vi "Day08-1.vi"() -> ()   [LabVIEW 2021]
panel:
  out "Numeric":i32
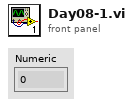
[diagram p1: front panel]
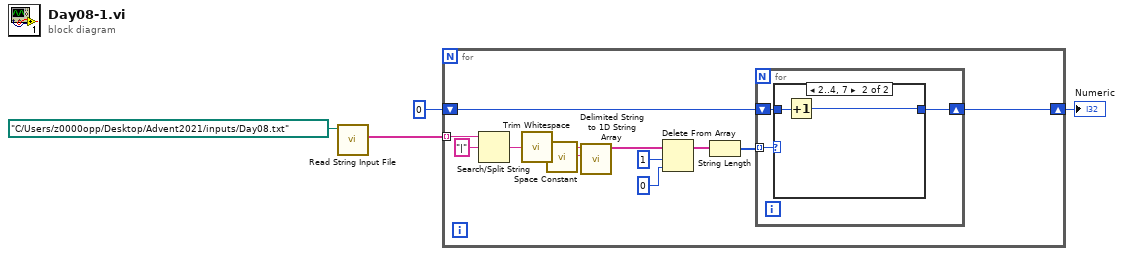
[diagram p0: block diagram]
diagram:
  n1 = call "Read String Input File.vi"("file path (dialog if empty)"=path "C:/Users/z0000opp/Desktop/Advent2021/inputs/Day08.txt") -> ("input values"=w3:string[])  [unwired: 10 in]
  n2 = for {
    tunnel: w3 -> [w16] mode=indexing
    shift-right: [w11] -> w1
    shift-left: 0 -> [w10]
    n3 = Search/Split String(string=w16, search string/char (-)="|") -> (match + rest of string=w9:string)  [unwired: 1 in, 2 out]
    n4 = call <vilib>:"Trim Whitespace.vi"("string"=w9) -> ("trimmed string"=w14:string)  [unwired: 1 in]
    n5 = call <vilib>:"Space Constant.vi"() -> ("String"=w13:string)
    n6 = call <vilib>:"Delimited String to 1D String Array.vi"("delimiter"=w13, "delimited string"=w14) -> ("string array"=w8:string[])  [unwired: 9 in]
    n7 = Delete From Array(array=w8, length=1, index=0) -> (array with subset deleted=w7:string[])  [unwired: 1 out]
    n8 = String Length(string=w7) -> (length=w12:i32[])
    n9 = for {
      tunnel: w12 -> [w19] mode=indexing
      shift-right: [w17] -> w11
      shift-left: w10 -> [w18]
      n10 = case shown="2..4, 7" w19 {
        tunnel: w18 -> [w20 w22]
        tunnel: [w20 w21] -> w17
        frame Default {
        }
        frame 2..4, 7 {
          n11 = Increment(x=w22) -> (x+1=w21:i32)
        }
      }
    }
  }
  "Numeric" <- w1
